vi "Open Shutter.vi"(8 "error in (no error)":errorcluster, 10 "Shutter to Open":T1=enum."Cy3 (532 nm)", 11 "Uniblitz Shutter in":refnum<class "Uniblitz Shutter.lvclass">) -> (0 "error out":errorcluster, 3 "Uniblitz Shutter out":refnum<class "Uniblitz Shutter.lvclass">)   [LabVIEW 2015, in "Uniblitz Shutter.lvlib" / "Uniblitz Shutter.lvclass"]
uses:
  Uniblitz Shutter.lvclass
  Resources/Type Defs/Excitation.ctl
  Uniblitz Shutter.lvclass/Uniblitz Shutter.ctl
  <vilib>/DAQmx/write.llb/DAQmx Write (Digital Bool 1Line 1Point).vi
  <vilib>/DAQmx/miscellaneous.llb/DAQmx Fill In Error Info.vi
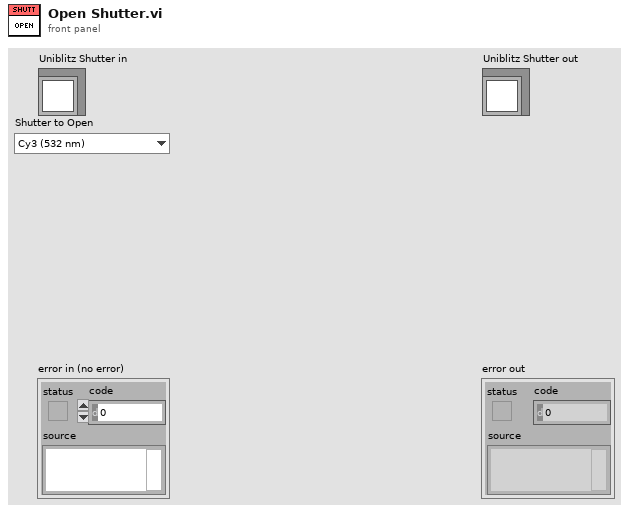
[diagram p1: front panel]
types:
  T1 = typedef "Excitation.ctl" = enum16{"Cy2 (473 nm)", "Cy3 (532 nm)", "Cy5 (639 nm)", "Cy7 (730 nm)", "Cy2/Cy3", "Cy3/Cy5", "Cy3/Cy7", "Cy5/Cy7"}
  T2 = cluster{"Excitation":T1, "DAQmx Channel":refnum<k21>, "Open?":bool}[]
  T3 = cluster{"Excitation":T1, "DAQmx Channel":refnum<k21>, "Open?":bool}
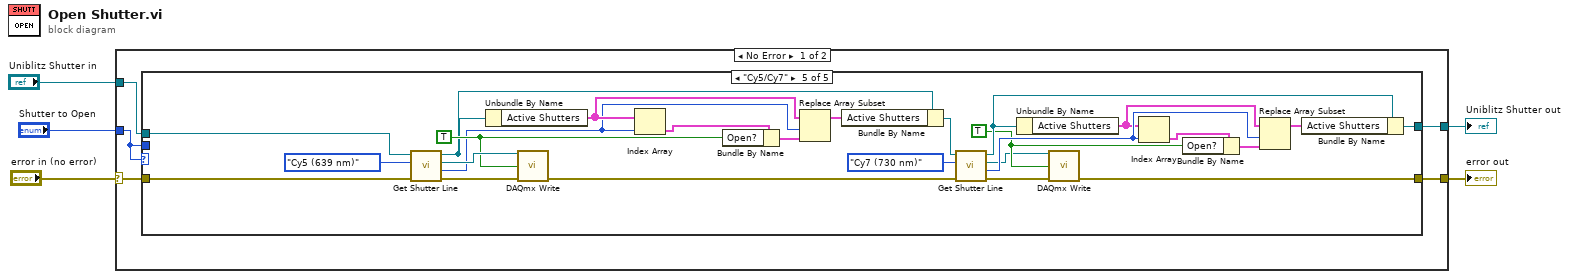
[diagram p0: block diagram]
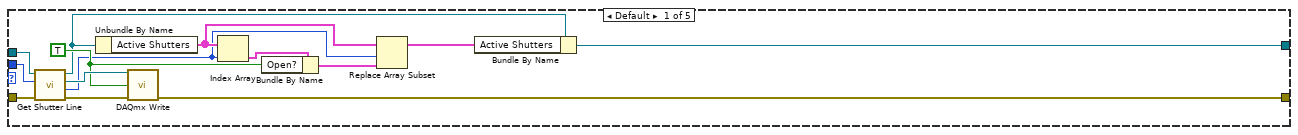
[diagram p2: hidden frame]
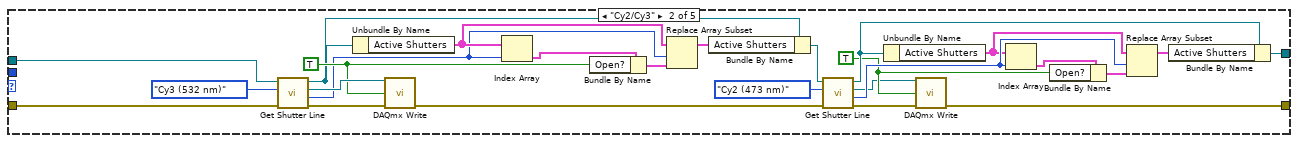
[diagram p3: hidden frame]
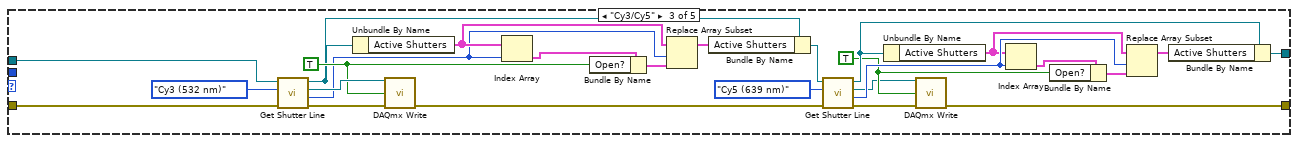
[diagram p4: hidden frame]
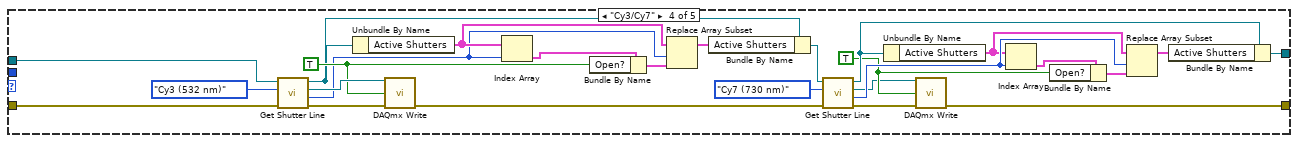
[diagram p5: hidden frame]
diagram:
  n1 = case shown="No Error" "error in (no error)" {
    selector: "error in (no error)" -> [w10 w130]
    tunnel: [w9 w130] -> w4
    tunnel: [w8 w129] -> w2
    tunnel: "Uniblitz Shutter in" -> [w7 w129]
    tunnel: "Shutter to Open" -> [w6 _]
    frame No Error {
      n2 = case shown="\"Cy5/Cy7\"" w6 {
        tunnel: w6 -> [w24 _ _ _ _]
        tunnel: w10 -> [w23 w50 w76 w102 w128]
        tunnel: [w20 w25 w51 w77 w103] -> w9
        tunnel: [w12 w27 w53 w79 w105] -> w8
        tunnel: w7 -> [w11 w40 w66 w92 w118]
        frame Default {
          w18 = TRUE ("data")
          n3 = call-dynamic "Get Shutter Line.vi"("error in (no error)"=w23, "Shutter"=w24, "Uniblitz Shutter in"=w11) -> ("error out"=w21:errorcluster, "Index"=w15:i32, "DAQmx Channel"=w22:refnum<k21>, "Uniblitz Shutter out"=w13:refnum<class "Uniblitz Shutter.lvclass">)  [unwired: 5 in]
          n4 = Unbundle By Name(w13) -> ("Active Shutters"=w17:T2)
          n5 = call-poly <vilib>:"DAQmx Write.vi"("task/channels in"=w22, "data"=w18, "error in"=w21) -> ("error out"=w20:errorcluster)  [unwired: 10 in, 2 out]
          n6 = Index Array(array=w17, index=w15) -> (element=w19:T3)
          n7 = Bundle By Name(cluster=w19, "Open?"=w18) -> (w16:T3)
          n8 = Replace Array Subset(array=w17, new element=w16, index=w15) -> (w14:T2)
          n9 = Bundle By Name(cluster=w13, "Active Shutters"=w14) -> (w12:refnum<class "Uniblitz Shutter.lvclass">)
        }
        frame "Cy2/Cy3" {
          w34 = TRUE ("data")
          w46 = TRUE ("data")
          n10 = call-dynamic "Get Shutter Line.vi"("error in (no error)"=w50, "Shutter"=Excitation."Cy3 (532 nm)", "Uniblitz Shutter in"=w40) -> ("error out"=w48:errorcluster, "Index"=w43:i32, "DAQmx Channel"=w49:refnum<k21>, "Uniblitz Shutter out"=w41:refnum<class "Uniblitz Shutter.lvclass">)  [unwired: 5 in]
          n11 = Unbundle By Name(w41) -> ("Active Shutters"=w45:T2)
          n12 = call-poly <vilib>:"DAQmx Write.vi"("task/channels in"=w49, "data"=w46, "error in"=w48) -> ("error out"=w26:errorcluster)  [unwired: 10 in, 2 out]
          n13 = Index Array(array=w45, index=w43) -> (element=w47:T3)
          n14 = Bundle By Name(cluster=w47, "Open?"=w46) -> (w44:T3)
          n15 = Replace Array Subset(array=w45, new element=w44, index=w43) -> (w42:T2)
          n16 = Bundle By Name(cluster=w41, "Active Shutters"=w42) -> (w28:refnum<class "Uniblitz Shutter.lvclass">)
          n17 = call-dynamic "Get Shutter Line.vi"("error in (no error)"=w26, "Shutter"=Excitation."Cy2 (473 nm)", "Uniblitz Shutter in"=w28) -> ("error out"=w32:errorcluster, "Index"=w37:i32, "DAQmx Channel"=w31:refnum<k21>, "Uniblitz Shutter out"=w39:refnum<class "Uniblitz Shutter.lvclass">)  [unwired: 5 in]
          n18 = Unbundle By Name(w39) -> ("Active Shutters"=w35:T2)
          n19 = call-poly <vilib>:"DAQmx Write.vi"("task/channels in"=w31, "data"=w34, "error in"=w32) -> ("error out"=w25:errorcluster)  [unwired: 10 in, 2 out]
          n20 = Index Array(array=w35, index=w37) -> (element=w33:T3)
          n21 = Bundle By Name(cluster=w33, "Open?"=w34) -> (w36:T3)
          n22 = Replace Array Subset(array=w35, new element=w36, index=w37) -> (w38:T2)
          n23 = Bundle By Name(cluster=w39, "Active Shutters"=w38) -> (w27:refnum<class "Uniblitz Shutter.lvclass">)
        }
        frame "Cy3/Cy5" {
          w60 = TRUE ("data")
          w72 = TRUE ("data")
          n24 = call-dynamic "Get Shutter Line.vi"("error in (no error)"=w76, "Shutter"=Excitation."Cy3 (532 nm)", "Uniblitz Shutter in"=w66) -> ("error out"=w74:errorcluster, "Index"=w69:i32, "DAQmx Channel"=w75:refnum<k21>, "Uniblitz Shutter out"=w67:refnum<class "Uniblitz Shutter.lvclass">)  [unwired: 5 in]
          n25 = Unbundle By Name(w67) -> ("Active Shutters"=w71:T2)
          n26 = call-poly <vilib>:"DAQmx Write.vi"("task/channels in"=w75, "data"=w72, "error in"=w74) -> ("error out"=w52:errorcluster)  [unwired: 10 in, 2 out]
          n27 = Index Array(array=w71, index=w69) -> (element=w73:T3)
          n28 = Bundle By Name(cluster=w73, "Open?"=w72) -> (w70:T3)
          n29 = Replace Array Subset(array=w71, new element=w70, index=w69) -> (w68:T2)
          n30 = Bundle By Name(cluster=w67, "Active Shutters"=w68) -> (w54:refnum<class "Uniblitz Shutter.lvclass">)
          n31 = call-dynamic "Get Shutter Line.vi"("error in (no error)"=w52, "Shutter"=Excitation."Cy5 (639 nm)", "Uniblitz Shutter in"=w54) -> ("error out"=w58:errorcluster, "Index"=w63:i32, "DAQmx Channel"=w57:refnum<k21>, "Uniblitz Shutter out"=w65:refnum<class "Uniblitz Shutter.lvclass">)  [unwired: 5 in]
          n32 = Unbundle By Name(w65) -> ("Active Shutters"=w61:T2)
          n33 = call-poly <vilib>:"DAQmx Write.vi"("task/channels in"=w57, "data"=w60, "error in"=w58) -> ("error out"=w51:errorcluster)  [unwired: 10 in, 2 out]
          n34 = Index Array(array=w61, index=w63) -> (element=w59:T3)
          n35 = Bundle By Name(cluster=w59, "Open?"=w60) -> (w62:T3)
          n36 = Replace Array Subset(array=w61, new element=w62, index=w63) -> (w64:T2)
          n37 = Bundle By Name(cluster=w65, "Active Shutters"=w64) -> (w53:refnum<class "Uniblitz Shutter.lvclass">)
        }
        frame "Cy3/Cy7" {
          w86 = TRUE ("data")
          w98 = TRUE ("data")
          n38 = call-dynamic "Get Shutter Line.vi"("error in (no error)"=w102, "Shutter"=Excitation."Cy3 (532 nm)", "Uniblitz Shutter in"=w92) -> ("error out"=w100:errorcluster, "Index"=w95:i32, "DAQmx Channel"=w101:refnum<k21>, "Uniblitz Shutter out"=w93:refnum<class "Uniblitz Shutter.lvclass">)  [unwired: 5 in]
          n39 = Unbundle By Name(w93) -> ("Active Shutters"=w97:T2)
          n40 = call-poly <vilib>:"DAQmx Write.vi"("task/channels in"=w101, "data"=w98, "error in"=w100) -> ("error out"=w78:errorcluster)  [unwired: 10 in, 2 out]
          n41 = Index Array(array=w97, index=w95) -> (element=w99:T3)
          n42 = Bundle By Name(cluster=w99, "Open?"=w98) -> (w96:T3)
          n43 = Replace Array Subset(array=w97, new element=w96, index=w95) -> (w94:T2)
          n44 = Bundle By Name(cluster=w93, "Active Shutters"=w94) -> (w80:refnum<class "Uniblitz Shutter.lvclass">)
          n45 = call-dynamic "Get Shutter Line.vi"("error in (no error)"=w78, "Shutter"=Excitation."Cy7 (730 nm)", "Uniblitz Shutter in"=w80) -> ("error out"=w84:errorcluster, "Index"=w89:i32, "DAQmx Channel"=w83:refnum<k21>, "Uniblitz Shutter out"=w91:refnum<class "Uniblitz Shutter.lvclass">)  [unwired: 5 in]
          n46 = Unbundle By Name(w91) -> ("Active Shutters"=w87:T2)
          n47 = call-poly <vilib>:"DAQmx Write.vi"("task/channels in"=w83, "data"=w86, "error in"=w84) -> ("error out"=w77:errorcluster)  [unwired: 10 in, 2 out]
          n48 = Index Array(array=w87, index=w89) -> (element=w85:T3)
          n49 = Bundle By Name(cluster=w85, "Open?"=w86) -> (w88:T3)
          n50 = Replace Array Subset(array=w87, new element=w88, index=w89) -> (w90:T2)
          n51 = Bundle By Name(cluster=w91, "Active Shutters"=w90) -> (w79:refnum<class "Uniblitz Shutter.lvclass">)
        }
        frame "Cy5/Cy7" {
          w112 = TRUE ("data")
          w124 = TRUE ("data")
          n52 = call-dynamic "Get Shutter Line.vi"("error in (no error)"=w128, "Shutter"=Excitation."Cy5 (639 nm)", "Uniblitz Shutter in"=w118) -> ("error out"=w126:errorcluster, "Index"=w121:i32, "DAQmx Channel"=w127:refnum<k21>, "Uniblitz Shutter out"=w119:refnum<class "Uniblitz Shutter.lvclass">)  [unwired: 5 in]
          n53 = Unbundle By Name(w119) -> ("Active Shutters"=w123:T2)
          n54 = call-poly <vilib>:"DAQmx Write.vi"("task/channels in"=w127, "data"=w124, "error in"=w126) -> ("error out"=w104:errorcluster)  [unwired: 10 in, 2 out]
          n55 = Index Array(array=w123, index=w121) -> (element=w125:T3)
          n56 = Bundle By Name(cluster=w125, "Open?"=w124) -> (w122:T3)
          n57 = Replace Array Subset(array=w123, new element=w122, index=w121) -> (w120:T2)
          n58 = Bundle By Name(cluster=w119, "Active Shutters"=w120) -> (w106:refnum<class "Uniblitz Shutter.lvclass">)
          n59 = call-dynamic "Get Shutter Line.vi"("error in (no error)"=w104, "Shutter"=Excitation."Cy7 (730 nm)", "Uniblitz Shutter in"=w106) -> ("error out"=w110:errorcluster, "Index"=w115:i32, "DAQmx Channel"=w109:refnum<k21>, "Uniblitz Shutter out"=w117:refnum<class "Uniblitz Shutter.lvclass">)  [unwired: 5 in]
          n60 = Unbundle By Name(w117) -> ("Active Shutters"=w113:T2)
          n61 = call-poly <vilib>:"DAQmx Write.vi"("task/channels in"=w109, "data"=w112, "error in"=w110) -> ("error out"=w103:errorcluster)  [unwired: 10 in, 2 out]
          n62 = Index Array(array=w113, index=w115) -> (element=w111:T3)
          n63 = Bundle By Name(cluster=w111, "Open?"=w112) -> (w114:T3)
          n64 = Replace Array Subset(array=w113, new element=w114, index=w115) -> (w116:T2)
          n65 = Bundle By Name(cluster=w117, "Active Shutters"=w116) -> (w105:refnum<class "Uniblitz Shutter.lvclass">)
        }
      }
    }
    frame Error {
    }
  }
  "error out" <- w4
  "Uniblitz Shutter out" <- w2
